vi "PSOC SHT40 Monitor.vi"() -> ()   [LabVIEW 2021]
doc: "This example performs writes and reads on a serial port, as directed by the user. You can press the Write and Read buttons, and change the Read Count, while the example is running.\n\nThe parameters set for the serial port must match the parameters of the connected instrument or device. In this example, the Read Count parameter specifies the number of bytes that the serial port reads. If there were more bytes at the port than the specified number, those bytes would not be read. If there were less bytes at the port than the specified number, you would receive a timeout error.\n\nThis example expands upon the flow control options for XON and XOFF, allowing the user to choose those control characters. Also, the user can enable or disable a termination character. Some devices require a termination character in order to identify the end of command strings. Some devices send a termination character to signify the end of data to be read. This example shows how you can end the Read operation once a termination character is detected in the buffer and/or append a termination character at the end of the Write data."
uses:
  Program Files (x86)/National Instruments/LabVIEW 2021/examples/Instrument IO/Serial/support/Serial - Settings.ctl
  Serial - XON-XOFF Characters.ctl
  Program Files (x86)/National Instruments/LabVIEW 2021/examples/Instrument IO/Serial/support/Serial - ASCII Characters.ctl
  <vilib>/Instr/_visa.llb/VISA Configure Serial Port (Instr).vi
  <vilib>/Analysis/NI_AALBase.lvlib
panel:
  out "Temperature Histogram":T1(graph)
  out "Temperature (deg C)":dbl(graph)
  in  "Termination Character":u8=13 format="%.0x"
  in  "End Write on Termination Character?":bool=TRUE
  in  "Stop":bool
  in  "Command":string="\n\n"
  out "Response":string
  in  "Write":bool
  in  "XON/XOFF Characters":T2={"XON"=enum."DC1", "XOFF"=enum."DC3"}
  in  "Serial Settings":T4={"baud rate"=115200, "data bits"=8, "parity"=enum."None", "stop bits"=10, "flow control"=0} {"flow control" items=["None"=0, "XON/XOFF"=1, "RTS/CTS"=2, "DTR/DSR"=4]; "stop bits" items=["1.0"=10, "1.5"=15, "2.0"=20]; "data bits" min=5 max=8 step=1; "baud rate" items=["75"=75, "110"=110, "134"=134, "150"=150, "300"=300, "600"=600, "1200"=1200, "1800"=1800, "2400"=2400, "4800"=4800, "7200"=7200, "9600"=9600, "14400"=14400, "19200"=19200, "28800"=28800, "38400"=38400, "56000"=56000, "57600"=57600, "115200"=115200, "128000"=128000, "230400"=230400]}
  in  "End Read on Termination Character?":bool=TRUE
  in  "VISA resource name":refnum<visa-resource-name>="COM7"
  # "Overview: Demonstrates the use of the VISA functions to write commands to and read responses from a serial instrument continuously in a loop.\nRequirements: NI-VISA Driver\nInstructions:\n1. Using Windows Device Manager take note of the COM port given by Windows to your microcontroller connection\n2. Change the VISA resource name to your COM port from step 1\n3. Run the VI.\n4. Press reset on your microcontroller\n5. Wait for the Ready to accept  Commands message\n6. The sample program response to Command :  T, A, B, I\n7. Specify a Command and click the Write button.\n8 The corresponding response should appear in the Response Window\n9. Click Stop to stop the VI."
  # "0xA is equivalent to a '\\n' character, which is a line feed."
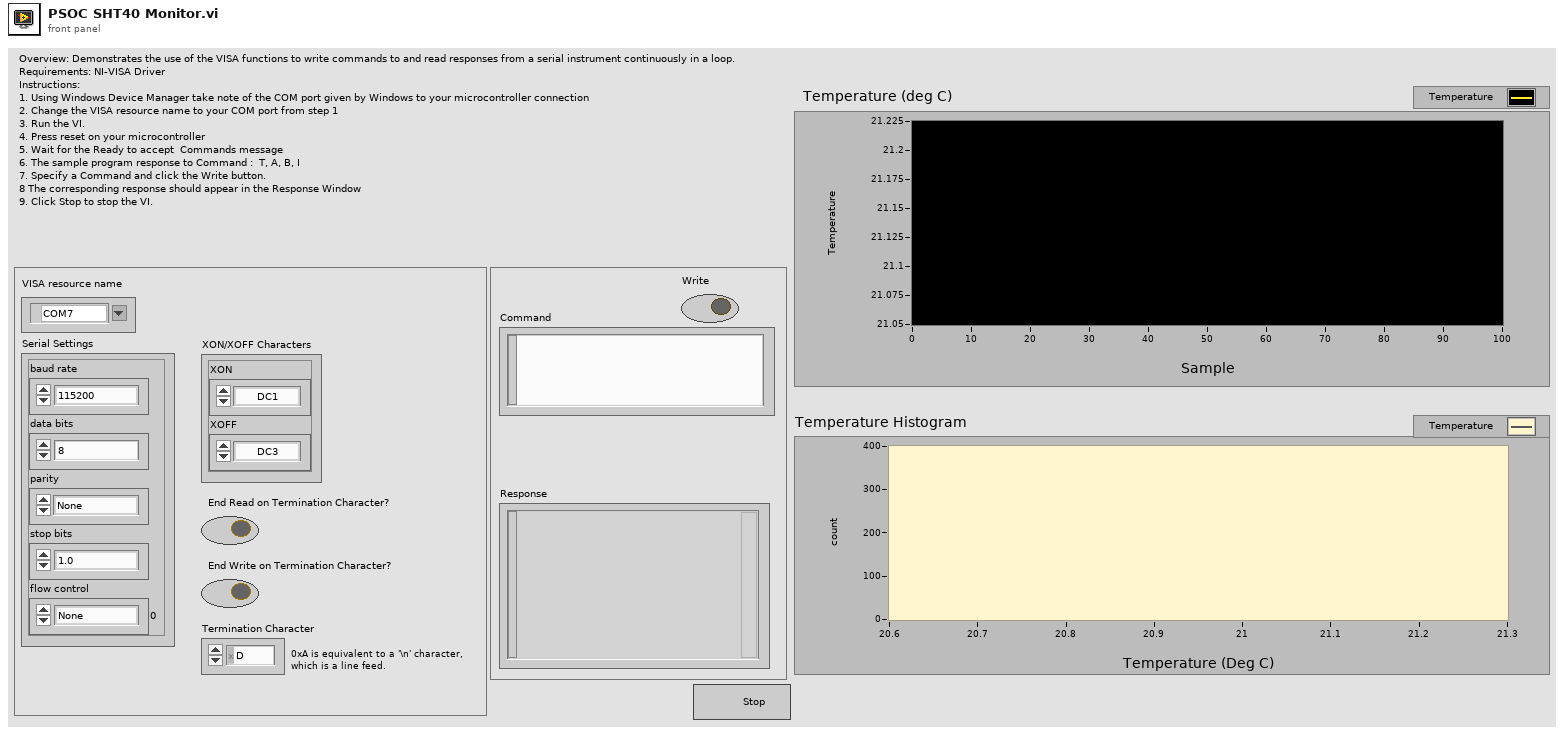
[diagram p1: front panel]
types:
  T1 = cluster{"X Values":dbl[], "Histogram: h(x)":i32[]}
  T2 = typedef "Serial - XON-XOFF Characters.ctl" = cluster{"XON":T3, "XOFF":T3}
  T3 = typedef "Serial - ASCII Characters.ctl" = enum16{"NUL", "SOH", "STX", "ETX", "EOT", "ENQ", "ACK", "BEL", "BS", "HT", "LF", "VT", "FF", "CR", "SO", "SI", "DLE", "DC1", "DC2", "DC3", "DC4", "NAK", "SYN", "ETB", "CAN", "EM", "SUB", "ESC", "FS", "GS", "RS", "US", "SP", "!", "\"", "#", "$", "%", "&", "'", "(", ")", "*", "+", ",", "- (-)", ".", "/", "0", "1", "2", "3", "4", "5", "6", "7", "8", "9", ":", ";", "<", "=", ">", "?", "@", "A", "B", "C", "D", "E", "F", "G", "H", "I", "J", "K", "L", "M", "N", "O", "P", "Q", "R", "S", "T", "U", "V", "W", "X", "Y", "Z", "[", "\\", "]", "^", "_", "`", "a", "b", "c", "d", "e", "f", "g", "h", "i", "j", "k", "l", "m", "n", "o", "p", "q", "r", "s", "t", "u", "v", "w", "x", "y", "z", "{", "|", "}", "~"}
  T4 = typedef "Serial - Settings.ctl" = cluster{"baud rate":u32, "data bits":u16, "parity":enum16{"None", "Odd", "Even", "Mark", "Space"}, "stop bits":u16, "flow control":u16}
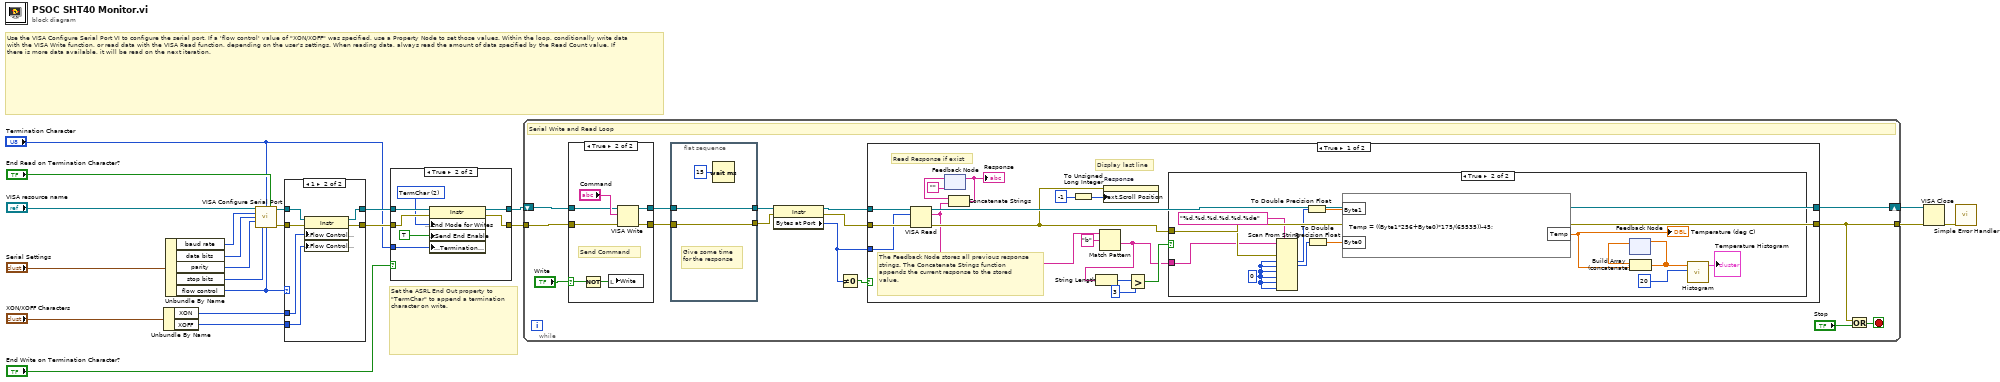
[diagram p0: block diagram]
diagram:
  # "Set the ASRL End Out property to \"TermChar\" to append a termination character on write."
  # "Use the VISA Configure Serial Port VI to configure the serial port. If a 'flow control' value of \"XON/XOFF\" was specified, use a Property Node to set those values. Within the loop, conditionally write data with the VISA Write function, or read data with the VISA Read function, depending on the user's settings. When reading data, always read the amount of data specified by the Read Count value. If there is more data available, it will be read on the next iteration."
  n1 = Unbundle By Name("XON/XOFF Characters") -> ("XON"=w8:T3, "XOFF"=w7:T3)
  n2 = Unbundle By Name("Serial Settings") -> ("baud rate"=w15:u32, "data bits"=w16:u16, "parity"=w17:enum16{"None", "Odd", "Even", "Mark", "Space"}, "stop bits"=w18:u16, "flow control"=w9:u16)
  n3 = call-poly "VISA Configure Serial Port"("VISA resource name"="VISA resource name", "termination char\n(0xA = '\\n' = LF)"="Termination Character", "Enable Termination\nChar (T)"="End Read on Termination Character?", "baud rate (9600)"=w15, "data bits (8)"=w16, "parity (0:none)"=w17, "stop bits (10: 1 bit)"=w18, "flow control (0:none)"=w9) -> ("VISA resource name out"=w19:refnum<visa-resource-name>, "error out"=w20:errorcluster)  [unwired: 2 in, 4 out]
  n4 = case shown="1" w9 {
    tunnel: [w23 w30] -> w6
    tunnel: [w24 w29] -> w4
    tunnel: w20 -> [w23 w28]
    tunnel: w19 -> [w24 w27]
    tunnel: w8 -> [_ w26]
    tunnel: w7 -> [_ w25]
    frame Default {
    }
    frame 1 {
      n5 = property class="Instr"(reference=w27, error in=w28, "Serial Settings:Flow Control XON Character"=w26, "Serial Settings:Flow Control XOFF Character"=w25) -> (reference out=w29:refnum<visa-resource-name>, error out=w30:errorcluster)
    }
  }
  n6 = case shown="True" "End Write on Termination Character?" {
    tunnel: w4 -> [w31 w39]
    tunnel: w6 -> [w32 w38]
    tunnel: [w31 w37] -> w3
    tunnel: [w32 w36] -> w5
    tunnel: "Termination Character" -> [_ w34]
    frame False {
    }
    frame True {
      w35 = u16 2 items=["None", "LastBit", "TermChar", "Break"] ("Serial Settings:Serial End Mode for Writes")
      n7 = property class="Instr"(reference=w39, error in=w38, "Serial Settings:End Mode for Writes"=w35, "Message Based Settings:Send End Enable"=TRUE, "Message Based Settings:Termination Character"=w34) -> (reference out=w37:refnum<visa-resource-name>, error out=w36:errorcluster)
    }
  }
  n8 = while {
    shift-right: [w54] -> w10
    shift-left: w3 -> [w53]
    tunnel: w5 -> [w52]
    tunnel: [w50] -> w11
    stop <- w51 stop-if-true
    # "Serial Write and Read Loop"
    n9 = case shown="True" "Write" {
      selector: "Write" -> [_ w61]
      tunnel: w53 -> [w59 w65]
      tunnel: w52 -> [w58 w64]
      tunnel: [w59 w63] -> w43
      tunnel: [w58 w62] -> w41
      frame False {
      }
      frame True {
        # "Send Command"
        n10 = Not(x=w61) -> (.not. x?=w60:bool)
        n11 = local write "Write"(w60) -> ()
        n12 = VISA Write(VISA resource name=w65, write buffer="Command", error in (no error)=w64) -> (VISA resource name out=w63:refnum<visa-resource-name>, error out=w62:errorcluster)  [unwired: 1 out]
      }
    }
    n13 = flat-sequence {
      tunnel: w43 -> [w57]
      tunnel: [w57] -> w42
      tunnel: w41 -> [w56]
      tunnel: [w56] -> w40
      frame #0 {
        # "Give some time\nfor the response"
        n14 = Wait (ms)(milliseconds to wait=u32 15) -> ()  [unwired: 1 out]
      }
    }
    n15 = property class="Instr"(reference=w42, error in=w40) -> (reference out=w46:refnum<visa-resource-name>, error out=w47:errorcluster, "Bytes at Port"=w44:u32)
    n16 = Not Equal To 0?(x=w44) -> (x != 0?=w45:bool)
    n17 = case shown="True" w45 {
      tunnel: [w76 w97] -> w54
      tunnel: w46 -> [w82 w97]
      tunnel: [w73 w96] -> w50
      tunnel: w47 -> [w81 w96]
      tunnel: w44 -> [w77 _]
      frame True {
        # "Read Response if exist"
        # "Display last line"
        # "The Feedback Node stores all previous response strings. The Concatenate Strings function appends the current response to the stored value."
        n18 = VISA Read(VISA resource name=w82, byte count=w77, error in (no error)=w81) -> (VISA resource name out=w76:refnum<visa-resource-name>, read buffer=w68:string, error out=w73:errorcluster)  [unwired: 1 out]
        n19 = feedback #1("") -> (w80:string)
        n20 = Concatenate Strings(w80, w68) -> (w79:string)
        "Response" <- w79
        n21 = feedback-in #1(w79) -> ()
        n22 = To Unsigned Long Integer(number=-1 ("Text.Scroll Position")) -> (unsigned 32bit integer=w74:u32)
        n23 = Match Pattern(string=w68, regular expression="b") -> (after substring=w67:string)  [unwired: 1 in, 3 out]
        n24 = String Length(string=w67) -> (length=w72:i32)
        n25 = property on="Response" class="Str"(error in=w73, "Text.Scroll Position"=w74) -> ()  [unwired: 1 in, 2 out]
        n26 = Greater?(x=w72, y=3) -> (0:w70:bool)
        n27 = case shown="True" w70 {
          tunnel: w73 -> [_ w94]
          tunnel: w67 -> [_ w92]
          frame False {
          }
          frame True {
            w95 = u8 0
            n28 = Scan From String(format string="%d,%d,%d,%d,%d,%de", input string=w92, error in=w94, default 1=w95, default 2=w95, default 3=w95, default 4=w95, default 5=w95, default 6=w95) -> (output 1=w91:u8, output 2=w90:u8)  [unwired: 5 in, 3 out]
            n29 = To Double Precision Float(number=w91) -> (double precision float=w89:dbl)
            n30 = To Double Precision Float(number=w90) -> (double precision float=w88:dbl)
            n31 = formula code="Temp = ((Byte1*256+Byte0)*175/(65535))-45;"("Byte1"=w89, "Byte0"=w88) -> ("Temp"=w87:dbl)
            "Temperature (deg C)" <- w87
            n32 = feedback #2() -> (w85:dbl[])  [unwired: 1 in]
            n33 = Build Array (concatenate)(w85, w87) -> (w86:dbl[])
            n34 = feedback-in #2(w86) -> ()
            n35 = call <vilib>:"Histogram.vi"("intervals"=20, "X"=w86) -> ("Histogram Graph"=→"Temperature Histogram":T1)  [unwired: 6 in, 3 out]
          }
        }
      }
      frame False {
      }
    }
    n36 = Or(x=w50, y="Stop") -> (x .or. y?=w51:bool)
  }
  n37 = VISA Close(VISA resource name=w10, error in (no error)=w11) -> (error out=w12:errorcluster)
  n38 = call <vilib>:"Simple Error Handler.vi"("error in (no error)"=w12) -> ()  [unwired: 1 in, 8 out]
